vi "createClassDataAndVersionsLUT.vi"(8 "error in":errorcluster, 9 "allClassNames":string[](array[string]), 10 "classHierarchyLUT":map{string, string[]}(c390)) -> (0 "error out":errorcluster, 1 "classPrivateDataLUT":map{string, variant[]}(c390), 2 "classVersionNumbersLUT":T1(c390), 4 "classPrivateDataLabelLUT":map{string, string[]}(c390))   [LabVIEW 2020, in "JKI JSON Object Serialization.lvlib" / "OOP_Utility.lvlib" / "Reflection.lvclass"]
doc: "GCraftsman JSON Object Serialization Toolkit\nwww.GCraftsman.com\nCopyright (c) 2017, GCraftsman"
uses:
  Reflection.lvclass
  Get Class Version from Type Descriptor.vi
  <vilib>/Utility/LVClass/Get LV Class Default Value By Name.vi
  Reflection.lvclass/Reflection.ctl
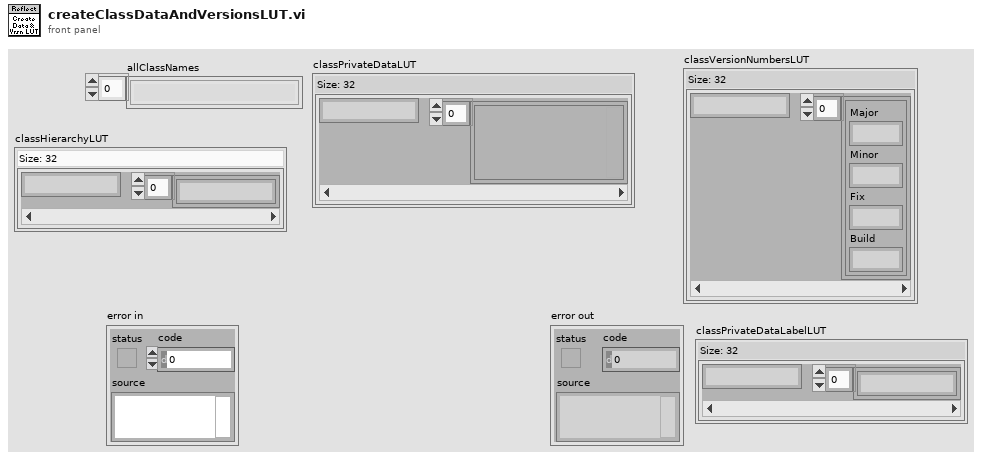
[diagram p1: front panel]
types:
  T1 = map{string, cluster{"Major":u16, "Minor":u16, "Fix":u16, "Build":u16}[]}
  T2 = cluster{"Major":u16, "Minor":u16, "Fix":u16, "Build":u16}
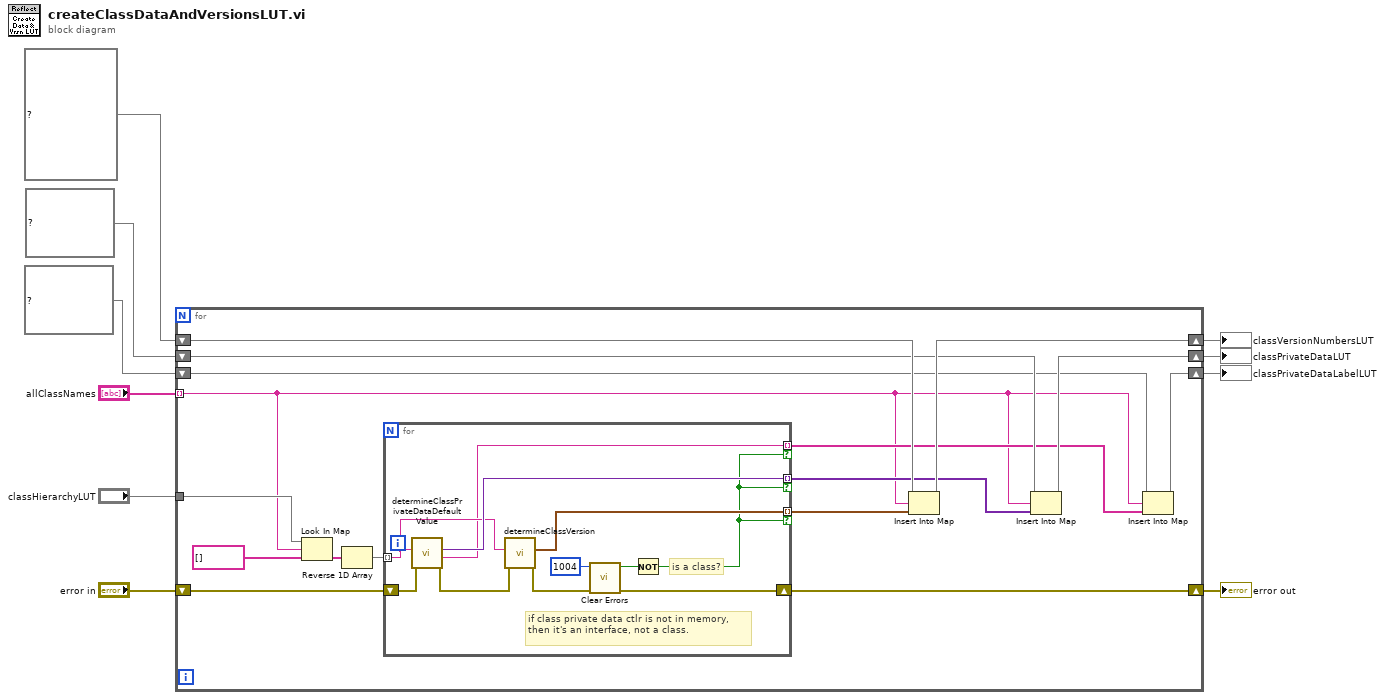
[diagram p0: block diagram]
diagram:
  n1 = for {
    tunnel: "allClassNames" -> [w17] mode=indexing
    shift-right: [w22] -> w8
    shift-left: T1 {} ("classHierarchyLUT") -> [w23]
    shift-right: [w20] -> w7
    shift-left: map{string, variant[]} {} ("classHierarchyLUT") -> [w21]
    shift-right: [w12] -> w5
    shift-left: "error in" -> [w11]
    tunnel: "classHierarchyLUT" -> [w25]
    shift-right: [w15] -> w4
    shift-left: map{string, string[]} {} ("classHierarchyLUT") -> [w16]
    n2 = Look In Map(map=w25, key=w17, default value=string[] [] ("classHierarchy")) -> (value=w24:string[])  [unwired: 1 out]
    n3 = Reverse 1D Array(array=w24) -> (reversed array=w13:string[])
    n4 = for {
      tunnel: w13 -> [w35] mode=indexing
      tunnel: [w36] -> w19 mode=indexing if=w27
      tunnel: [w34] -> w14 mode=indexing if=w27
      shift-right: [w30] -> w12
      shift-left: w11 -> [w33]
      tunnel: [w32] -> w18 mode=indexing if=w27
      # "is a class?"
      # "if class private data ctlr is not in memory, then it's an interface, not a class."
      n5 = call "determineClassPrivateDataDefaultValue.vi"("error in (no error)"=w33, "className"=w35) -> ("error out"=w37:errorcluster, "privateDataClusterLabel"=w32:string, "privateDataDefaultValue"=w36:variant)  [unwired: 7 in]
      n6 = call "determineClassVersion.vi"("error in (no error)"=w37, "className"=w35) -> ("error out"=w31:errorcluster, "Version"=w34:T2)  [unwired: 8 in]
      n7 = call <vilib>:"Clear Errors.vi"("error in (no error)"=w31, "specific error code to clear (0: all)"=1004) -> ("error out"=w30:errorcluster, "specific error cleared?"=w28:bool)  [unwired: 4 in]
      n8 = Not(x=w28) -> (.not. x?=w27:bool)
    }
    n9 = Insert Into Map(map in=w23, key=w17, value=w14) -> (map out=w22:T1)  [unwired: 2 out]
    n10 = Insert Into Map(map in=w21, key=w17, value=w19) -> (map out=w20:map{string, variant[]})  [unwired: 2 out]
    n11 = Insert Into Map(map in=w16, key=w17, value=w18) -> (map out=w15:map{string, string[]})  [unwired: 2 out]
  }
  "error out" <- w5
  "classVersionNumbersLUT" <- w8
  "classPrivateDataLUT" <- w7
  "classPrivateDataLabelLUT" <- w4
